vi "get channels.vi"(11 "Increment configuration in":refnum<class "Increment configuration.lvclass">) -> (2 "channels":refnum<class "TBM channel.lvclass">[](array[class]), 3 "Increment configuration out":refnum<class "Increment configuration.lvclass">)   [LabVIEW 2015, in "Increment configuration.lvclass"]
doc: "Returns an array of all Channels currently added to this configuration object."
uses:
  Increment configuration.lvclass
  <vilib>/NI/Tag Bus Module Framework/channel/TBM channel.lvclass
  Increment configuration.lvclass/Increment configuration.ctl
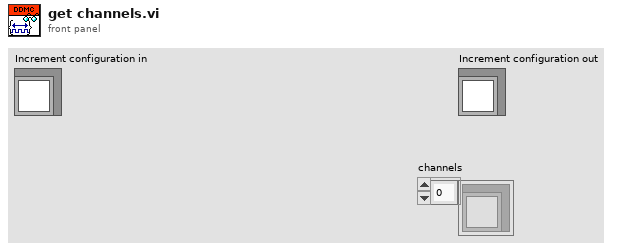
[diagram p1: front panel]
types:
  T1 = typedef "Increment configuration.lvclass/Line.ctl" = cluster{"Name":string, "channel in":refnum<class "TBM channel.lvclass">, "channel out":refnum<class "TBM channel.lvclass">}
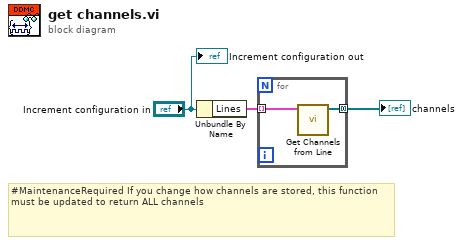
[diagram p0: block diagram]
diagram:
  # "#MaintenanceRequired If you change how channels are stored, this function must be updated to return ALL channels"
  n1 = Unbundle By Name("Increment configuration in") -> ("Lines"=w2:T1[])
  n2 = for {
    tunnel: w2 -> [w5] mode=indexing
    tunnel: [w4] -> w1 mode=concatenating
    n3 = call "Get Channels from Line.vi"("Line"=w5) -> ("Channels"=w4:refnum<class "TBM channel.lvclass">[])  [unwired: 10 in]
  }
  "channels" <- w1
  "Increment configuration out" <- "Increment configuration in"
